vi "Set Rate.vi"(8 "error in (no error)":errorcluster, 10 "Rate":dbl, 11 "Elevator in":refnum<class "Elevator.lvclass">) -> (0 "error out":errorcluster, 3 "Elevator out":refnum<class "Elevator.lvclass">)   [LabVIEW 2014, in "Elevator.lvlib" / "Elevator.lvclass"]
uses:
  Elevator.lvclass
  Elevator Messages/Current Motors with Encoder State Msg/Current Motors with Encoder State Msg.lvclass
  Elevator.lvclass/Elevator.ctl
  Motor with Encoders/Motors with Encoders Messages/Set Rate Msg/Set Rate  (RPM) Msg.lvclass/Set Rate  (RPM) Msg.ctl
  <vilib>/ActorFramework/Message Enqueuer/Message Enqueuer.lvclass/Message Enqueuer.ctl
  <vilib>/ActorFramework/Actor/Actor.lvclass/Actor.ctl
  <vilib>/ActorFramework/Message Enqueuer/Enqueue.vi
  <vilib>/ActorFramework/Message Enqueuer/Init from Existing Queue.vi
  <vilib>/ActorFramework/Message Priority Queue/Priority Enqueue.vi
  Motor with Encoders/Motors with Encoders Messages/Set Rate Msg/Set Rate  (RPM) Msg.lvclass
  <vilib>/ActorFramework/Message Enqueuer/Message Enqueuer.lvclass
  Motor with Encoders/Motors with Encoders Messages/Request Motors with Encoders State Msg/Request Motors with Encoders State Msg.lvclass
  <vilib>/ActorFramework/Actor/Actor.lvclass
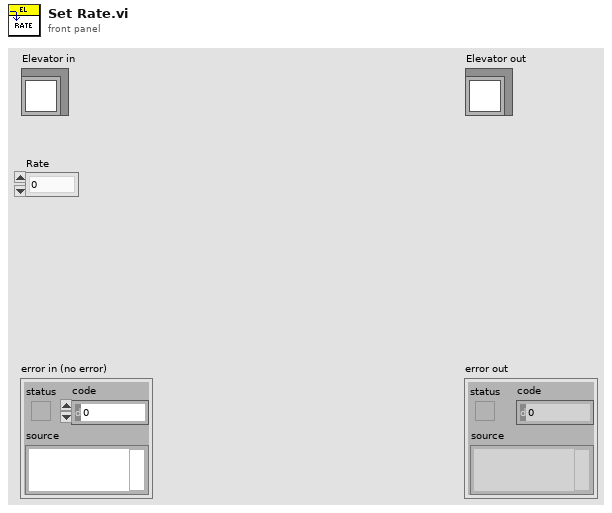
[diagram p1: front panel]
types:
  T1 = enum16{"Critical", "Error", "Warning", "Informational", "Debug"}
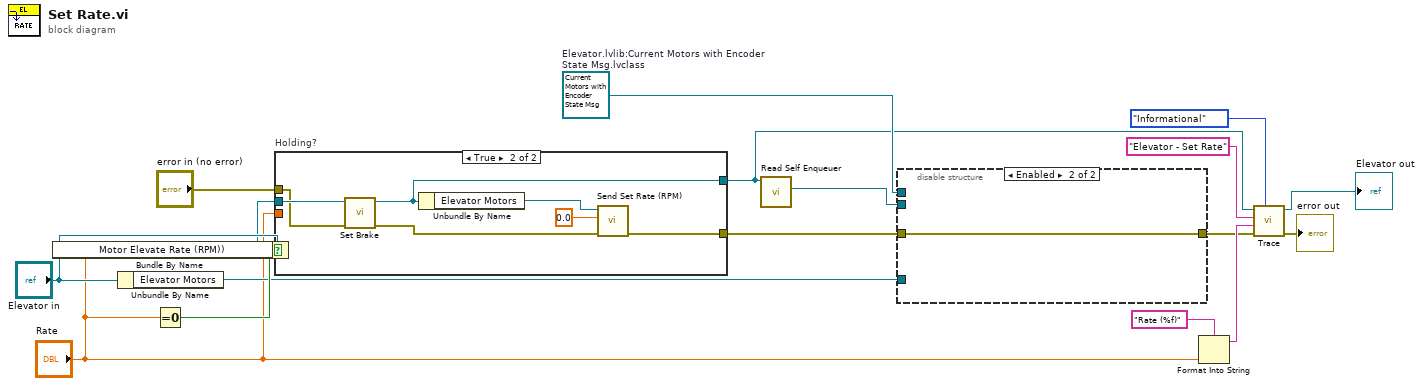
[diagram p0: block diagram]
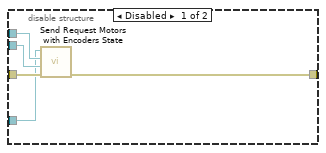
[diagram p2: hidden frame]
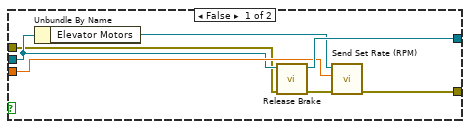
[diagram p3: hidden frame]
diagram:
  w9 = refnum<class "Current Motors with Encoder State Msg.lvclass"> refnum  # Elevator.lvlib:Current Motors with Encoder State Msg.lvclass
  n1 = Bundle By Name(cluster="Elevator in", "Motor Elevate Rate (RPM))"="Rate") -> (w2:refnum<class "Elevator.lvclass">)
  n2 = Unbundle By Name("Elevator in") -> ("Elevator Motors"=w4:refnum<class "Message Enqueuer.lvclass">)
  n3 = Equal To 0?(x="Rate") -> (x = 0?=w8:bool)
  n4 = case "Holding?" shown="True" w8 {
    tunnel: w2 -> [w21 w31]
    tunnel: [w24 w29] -> w7
    tunnel: "error in (no error)" -> [w20 w30]
    tunnel: [w18 w25] -> w6
    tunnel: "Rate" -> [w22 _]
    frame False {
      n5 = Unbundle By Name(w21) -> ("Elevator Motors"=w23:refnum<class "Message Enqueuer.lvclass">)
      n6 = call-dynamic "Release Brake.vi"("error in (no error)"=w20, "Elevator in"=w21) -> ("error out"=w19:errorcluster, "Elevator out"=w24:refnum<class "Elevator.lvclass">)  [unwired: 8 in]
      n7 = call "Send Set Rate (RPM).vi"("error in (no error)"=w19, "Rate (RPM)"=w22, "Message Enqueuer"=w23) -> ("error out"=w18:errorcluster)  [unwired: 7 in, 1 out]
    }
    frame True {
      n8 = call-dynamic "Set Brake.vi"("error in (no error)"=w30, "Elevator in"=w31) -> ("error out"=w26:errorcluster, "Elevator out"=w29:refnum<class "Elevator.lvclass">)  [unwired: 8 in]
      n9 = Unbundle By Name(w29) -> ("Elevator Motors"=w28:refnum<class "Message Enqueuer.lvclass">)
      n10 = call "Send Set Rate (RPM).vi"("error in (no error)"=w26, "Rate (RPM)"=0.0, "Message Enqueuer"=w28) -> ("error out"=w25:errorcluster)  [unwired: 7 in, 1 out]
    }
  }
  n11 = call <vilib>:"Read Self Enqueuer.vi"("Actor"=w7) -> ("Self Enqueuer"=w10:refnum<class "Message Enqueuer.lvclass">)  [unwired: 10 in]
  n12 = disable-structure shown="Enabled" {
    disable-tunnel: [w36 w37] -> w11
    disable-tunnel: w10 -> [w35 _]
    disable-tunnel: w9 -> [w34 _]
    disable-tunnel: w6 -> [w33 w37]
    disable-tunnel: w4 -> [w32 _]
    frame Disabled {
      n13 = call "Send Request Motors with Encoders State.vi"("error in (no error)"=w33, "Requestor Queue"=w35, "Current State Msg"=w34, "Message Enqueuer"=w32) -> ("error out"=w36:errorcluster)  [unwired: 6 in, 1 out]
    }
    frame Enabled {
    }
  }
  n14 = Format Into String(format string="Rate (%f)", "Rate") -> (resulting string=w15:string)  [unwired: 2 in, 1 out]
  n15 = call-dynamic "Trace.vi"("Trace Level"=T1."Informational", "error in (no error)"=w11, "System Message"=w15, "System Action"="Elevator - Set Rate", "System Actor in"=w7) -> ("error out"=→"error out":errorcluster, "System Actor out"=→"Elevator out":refnum<class "Elevator.lvclass">)  [unwired: 5 in]
